vi "TCL Get Base Fragments - 1event1frag.vi"(3 "error in (no error)":errorcluster, 4 "fragment":string, 5 "event number":i32) -> (0 "error out":errorcluster, 1 "values":string[][](array[string]), 2 "fragments out":string[](array[string]))   [LabVIEW 2010]
uses:
  TCL Global.vi
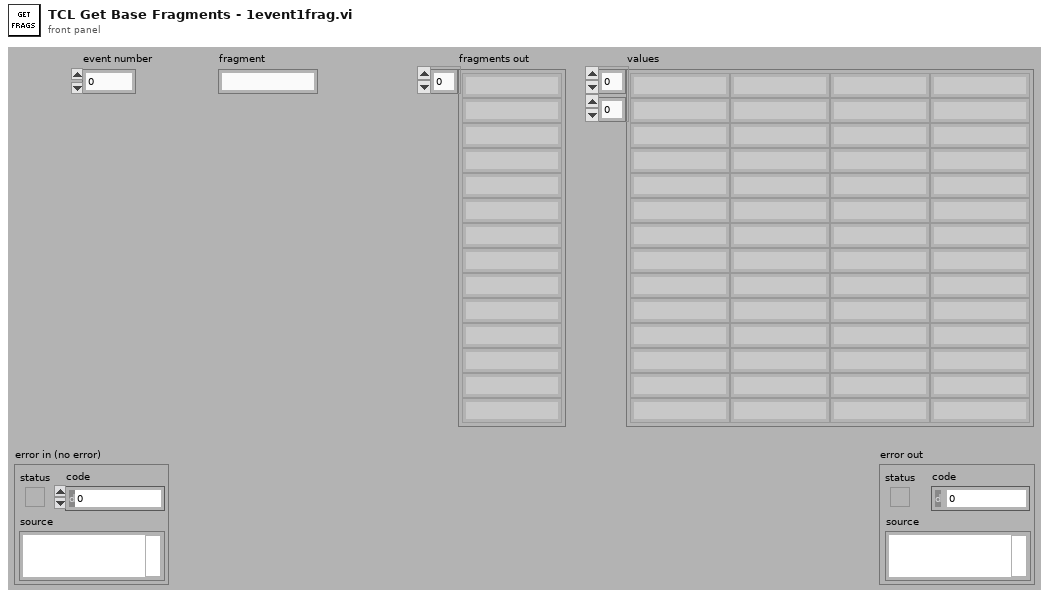
[diagram p1: front panel]
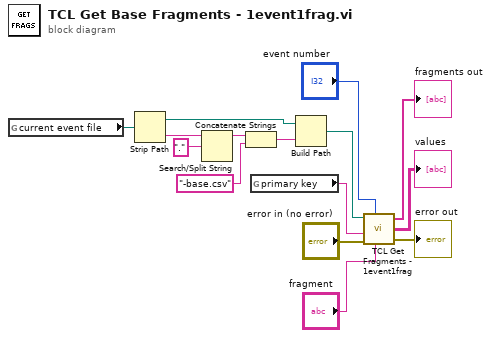
[diagram p0: block diagram]
diagram:
  n1 = global read "TCL Global.vi" "current event file"() -> (w8:path)
  n2 = Strip Path(path=w8) -> (stripped path=w4:path, name=w7:string)
  n3 = Search/Split String(string=w7, search string/char (-)=".") -> (substring before match=w5:string)  [unwired: 1 in, 2 out]
  n4 = Concatenate Strings(w5, "-base.csv" ("string")) -> (w3:string)
  n5 = global read "TCL Global.vi" "primary key"() -> (w9:string)
  n6 = Build Path(base path=w4, name or relative path=w3) -> (appended path=w2:path)
  n7 = call "TCL Get Fragments - 1event1frag.vi"("event file"=w2, "event number"="event number", "primary key"=w9, "fragment"="fragment", "error in (no error)"="error in (no error)") -> ("fragments out"=→"fragments out":string[], "values"=→"values":string[][], "error out"=→"error out":errorcluster)  [unwired: 1 in]
